vi "Initialize.vi"(7 "Serial Configuration":T1={"Baud Rate"=576000, "Parity"=0, "Data Bits"=7, "Stop Bits"=10, "Flow Control"=0} {"Flow Control" items=["None", "XON/XOFF", "RTS/CTS", "XON/XOFF & RTS/CTS", "DTR/DSR", "XON/XOFF & DTR/DSR"]; "Stop Bits" items=["1.0"=10, "1.5"=15, "2.0"=20]; "Data Bits" items=["7"=7, "8"=8]; "Parity" items=["None", "Odd", "Even", "Mark", "Space"]; "Baud Rate" items=["300"=300, "600"=600, "1200"=1200, "2400"=2400, "4800"=4800, "9600"=9600, "19200"=19200]}, 8 "error in (no error)":errorcluster, 9 "Reset (True)":bool=TRUE, 10 "ID Query (True)":bool=TRUE, 11 "VISA resource name":refnum<visa-resource-name>) -> (0 "error out":errorcluster, 3 "VISA resource name out":refnum<visa-resource-name>)   [LabVIEW 2020, in "BDAQ-6104.lvlib"]
doc: "Establishes communication with the instrument and optionally performs an instrument identification query and/or an instrument reset. It also places the instrument in a default state needed for other instrument driver operations. Therefore, call this VI before calling other instrument driver VIs for this instrument. Generally, you need to call the <b>Initialize</b> VI only once at the beginning of an application."
uses:
  <instrlib>/BDAQ-6104/BDAQ-6104.lvlib
panel:
  # "(c) 2014 <Enter Company Name Here>.  ALL RIGHTS RESERVED."
  # "EDIT: Serial settings must match those on the physical instrument.  Review user's manual to determine the correct Flow Control protocol for the instrument.  \"None\" is the least robust option for this setting, and could lead to unreliable data transmission."
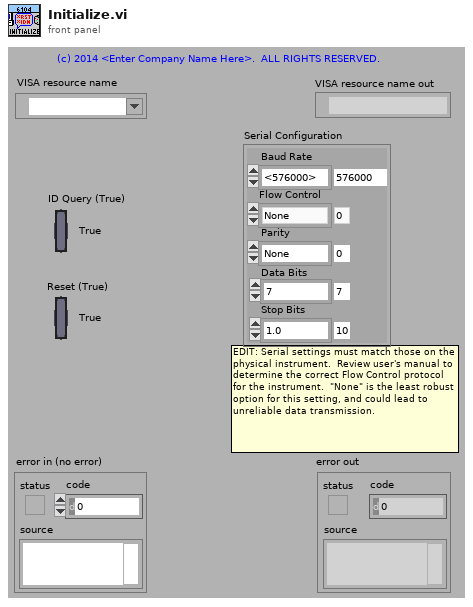
[diagram p1: front panel]
types:
  T1 = cluster{"Baud Rate":u32, "Parity":u16, "Data Bits":u16, "Stop Bits":u16, "Flow Control":u16}
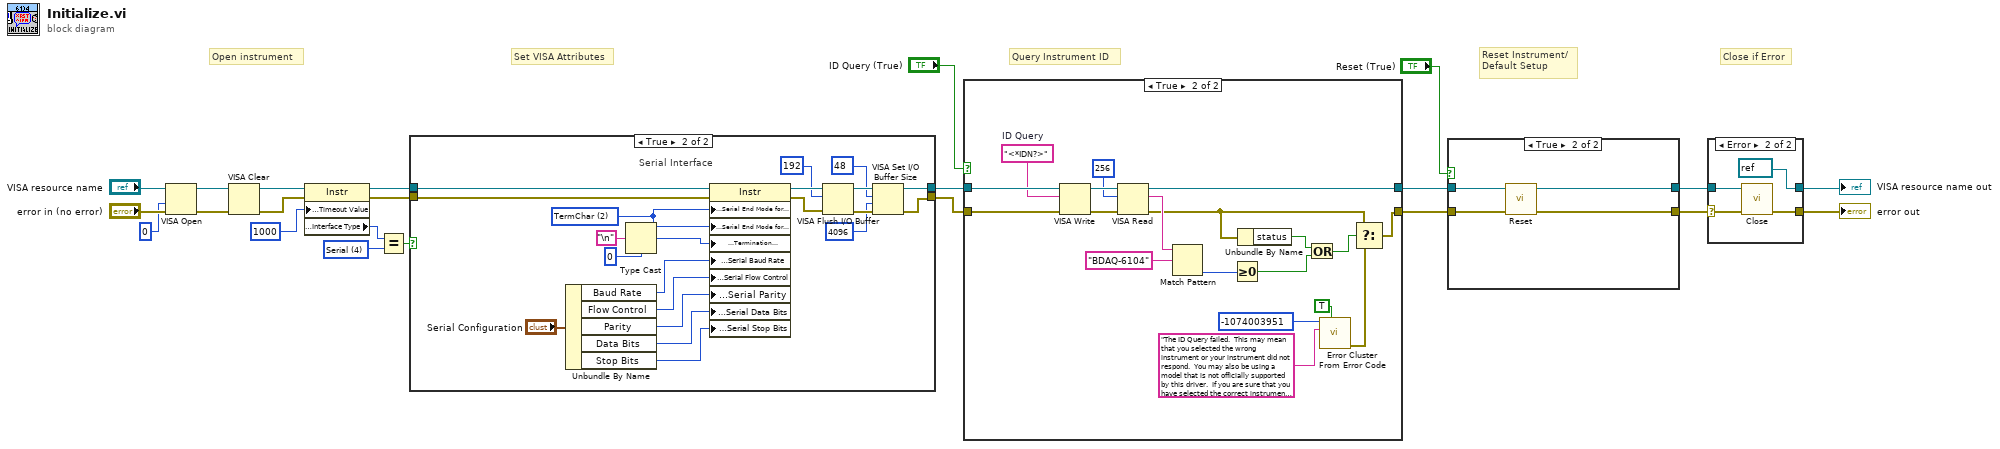
[diagram p0: block diagram]
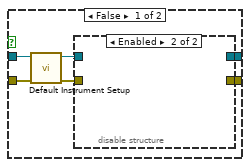
[diagram p4: hidden frame]
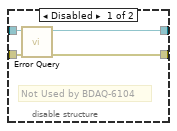
[diagram p5: hidden frame]
diagram:
  w10 = u16 4 items=["Serial"=4] ("Interface Information:Interface Type")
  # "Set VISA Attributes"
  # "Close if Error"
  # "Query Instrument ID"
  # "Reset Instrument/\nDefault Setup"
  # "Open instrument"
  n1 = VISA Open(access mode=u32 0, error in (no error)="error in (no error)", VISA resource name="VISA resource name") -> (VISA resource name=w8:refnum<visa-resource-name>, error out=w7:errorcluster)  [unwired: 2 in]
  n2 = VISA Clear(VISA resource name=w8, error in (no error)=w7) -> (VISA resource name out=w6:refnum<visa-resource-name>, error out=w5:errorcluster)
  n3 = property class="Instr"(reference=w6, error in=w5, "General Settings:Timeout Value"=u32 1000) -> (reference out=w13:refnum<visa-resource-name>, error out=w12:errorcluster, "Interface Information:Interface Type"=w17:u16)
  n4 = Equal?(x=w17, y=w10) -> (x = y?=w11:bool)
  n5 = case shown="True" w11 {
    tunnel: [w24 w43] -> w15
    tunnel: [w25 w40] -> w14
    tunnel: w13 -> [w24 w45]
    tunnel: w12 -> [w25 w46]
    frame False {
      # "Only serial is supported by the BDAQ-6104"
    }
    frame True {
      w33 = u16 2 items=["None", "LastBit", "TermChar"] ("Serial Settings:Serial End Mode for Reads")
      # "Serial Interface"
      n6 = Unbundle By Name("Serial Configuration") -> ("Baud Rate"=w31:u32, "Flow Control"=w27:u16, "Parity"=w29:u16, "Data Bits"=w30:u16, "Stop Bits"=w26:u16)
      n7 = Type Cast(type=u8 0, x="\n" ("Line Feed Constant")) -> (*(type *) &x=w32:u8)
      n8 = property class="Instr"(reference=w45, error in=w46, "Serial Settings:Serial End Mode for Reads"=w33, "Serial Settings:Serial End Mode for Writes"=w33, "Message Based Settings:Termination Character"=w32, "Serial Settings:Serial Baud Rate"=w31, "Serial Settings:Serial Flow Control"=w27, "Serial Settings:Serial Parity"=w29, "Serial Settings:Serial Data Bits"=w30, "Serial Settings:Serial Stop Bits"=w26) -> (reference out=w39:refnum<visa-resource-name>, error out=w42:errorcluster)
      n9 = VISA Flush I/O Buffer(VISA resource name=w39, mask (16)=u16 192, error in (no error)=w42) -> (VISA resource name out=w44:refnum<visa-resource-name>, error out=w41:errorcluster)
      n10 = VISA Set I/O Buffer Size(VISA resource name=w44, mask (16)=u16 48, size (4096)=u32 4096 ("size (0)"), error in (no error)=w41) -> (VISA resource name out=w43:refnum<visa-resource-name>, error out=w40:errorcluster)
    }
  }
  n11 = case shown="True" "ID Query (True)" {
    tunnel: [w47 w67] -> w22
    tunnel: [w48 w64] -> w23
    tunnel: w15 -> [w48 w65]
    tunnel: w14 -> [w47 w66]
    frame False {
    }
    frame True {
      w58 = "<*IDN?>"  # ID Query
      n12 = VISA Write(VISA resource name=w65, write buffer=w58, error in (no error)=w66) -> (VISA resource name out=w62:refnum<visa-resource-name>, error out=w61:errorcluster)  [unwired: 1 out]
      n13 = VISA Read(VISA resource name=w62, byte count=u32 256, error in (no error)=w61) -> (VISA resource name out=w64:refnum<visa-resource-name>, read buffer=w63:string, error out=w52:errorcluster)  [unwired: 1 out]
      n14 = Match Pattern(string=w63, regular expression="BDAQ-6104") -> (offset past match=w53:i32)  [unwired: 1 in, 3 out]
      n15 = Greater Or Equal To 0?(x=w53) -> (x >= 0?=w50:bool)
      n16 = Unbundle By Name(w52) -> ("status"=w51:bool)
      n17 = Or(x=w51, y=w50) -> (x .or. y?=w49:bool)
      n18 = call <vilib>:"Error Cluster From Error Code.vi"("show call chain? (False)"=TRUE, "error message (\"\")"="The ID Query failed.  This may mean that you selected the wrong instrument or your instrument did not respond.  You may also be using a model that is not officially supported by this driver.  If you are sure that you have selected the correct instrument and it is responding, try disabling the ID Query." ("Source (VI Name)"), "error code (0)"=-1074003951 ("Code")) -> ("error out"=w57:errorcluster)  [unwired: 6 in]
      n19 = Select(t=w52, s=w49, f=w57) -> (s? t:f=w67:errorcluster)
    }
  }
  n20 = case shown="True" "Reset (True)" {
    tunnel: w22 -> [w72 w78]
    tunnel: [w69 w81] -> w1
    tunnel: w23 -> [w73 w79]
    tunnel: [w70 w80] -> w2
    frame False {
      n21 = call <instrlib>:"Default Instrument Setup.vi"("error in (no error)"=w72, "VISA resource name"=w73) -> ("error out"=w68:errorcluster, "VISA resource name out"=w71:refnum<visa-resource-name>)  [unwired: 8 in]
      n22 = disable-structure shown="Enabled" {
        disable-tunnel: w71 -> [w77 _]
        disable-tunnel: [w76 _] -> w70
        disable-tunnel: [w75 _] -> w69
        disable-tunnel: w68 -> [w74 _]
        frame Disabled {
          # "Not Used by BDAQ-6104"
          n23 = call <instrlib>:"Error Query.vi"("error in (no error)"=w74, "VISA resource name"=w77) -> ("error out"=w75:errorcluster, "VISA resource name out"=w76:refnum<visa-resource-name>)  [unwired: 6 in, 2 out]
        }
        frame Enabled {
        }
      }
    }
    frame True {
      n24 = call <instrlib>:"Reset.vi"("error in (no error)"=w78, "VISA resource name"=w79) -> ("error out"=w81:errorcluster, "VISA resource name out"=w80:refnum<visa-resource-name>)  [unwired: 8 in]
    }
  }
  n25 = case shown="Error" w1 {
    selector: w1 -> [w82 w85]
    tunnel: w2 -> [w83 w86]
    tunnel: [w83 refnum<visa-resource-name> refnum ("VISA resource name out")] -> w4
    tunnel: [w82 w87] -> w3
    frame No Error {
    }
    frame Error {
      n26 = call <instrlib>:"Close.vi"("error in (no error)"=w85, "VISA resource name"=w86) -> ("error out"=w87:errorcluster)  [unwired: 9 in]
    }
  }
  "VISA resource name out" <- w4
  "error out" <- w3
